vi "Read issued_at.vi"(8 "error in (no error)":errorcluster, 11 "Oauth2.Salesforce in":refnum<class "Oauth2.Salesforce.lvclass">) -> (0 "error out":errorcluster, 2 "issued_at":timestamp, 3 "Oauth2.Salesforce out":refnum<class "Oauth2.Salesforce.lvclass">)   [LabVIEW 2017, in "Oauth2.Salesforce.lvclass"]
uses:
  Oauth2.Salesforce.lvclass
  Oauth2.Salesforce.lvclass/Oauth2.Salesforce.ctl
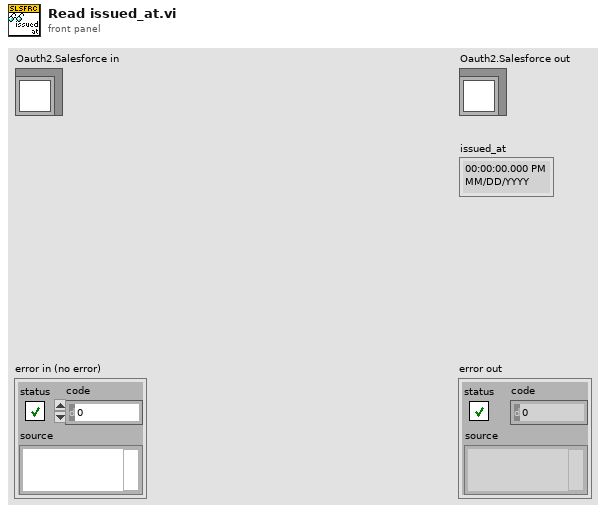
[diagram p1: front panel]
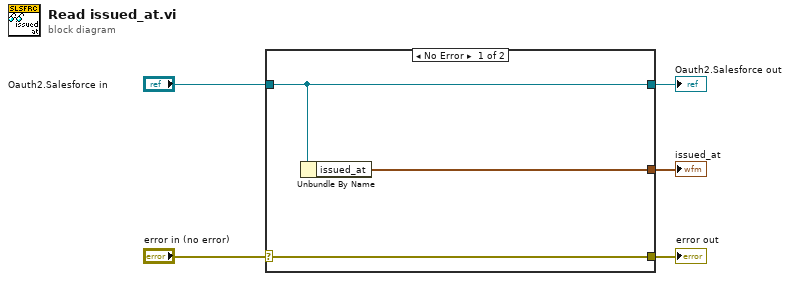
[diagram p0: block diagram]
diagram:
  n1 = case shown="No Error" "error in (no error)" {
    selector: "error in (no error)" -> [w8 w9]
    tunnel: [w8 w9] -> w4
    tunnel: [w7 w10] -> w2
    tunnel: "Oauth2.Salesforce in" -> [w7 w10]
    tunnel: [w6 _] -> w1
    frame No Error {
      n2 = Unbundle By Name(w7) -> ("issued_at"=w6:timestamp)
    }
    frame Error {
    }
  }
  "error out" <- w4
  "Oauth2.Salesforce out" <- w2
  "issued_at" <- w1
